vi "Handle setConfiguration.vi"(8 "error in (no error)":errorcluster, 10 "setConfiguration":variant, 11 "Inst.RP100 in":refnum<class "Inst.RP100.lvclass">) -> (0 "error out":errorcluster, 3 "Inst.RP100 out":refnum<class "Inst.RP100.lvclass">)   [LabVIEW 2019, in "Inst.RP100.lvclass"]
uses:
  Inst.RP100.lvclass
  45e4b271-6884-462c-ad3a-d505ab08eb62.vi
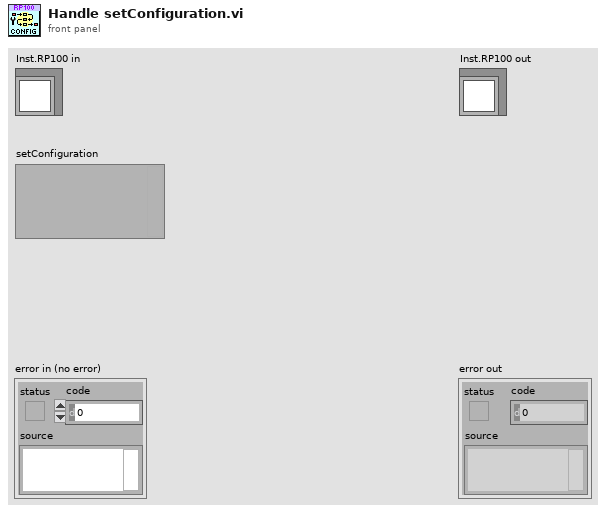
[diagram p1: front panel]
types:
  T1 = typedef "Inst.RP100.lvclass/Inst.RP100.Configuration--Cluster.ctl" = cluster{"Example Setting 1":dbl, "Example Setting 2":dbl, "Example Setting 3":string}
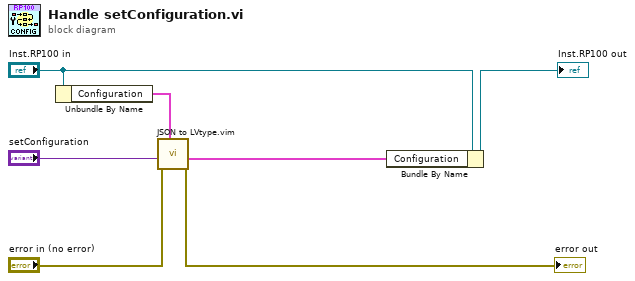
[diagram p0: block diagram]
diagram:
  n1 = Unbundle By Name("Inst.RP100 in") -> ("Configuration"=w6:T1)
  n2 = call "JSON to LVtype.vim"("type"=w6, "error in (no error)"="error in (no error)", "JSON Data in"="setConfiguration") -> ("error out"=→"error out":errorcluster, "Data out"=w1:T1)  [unwired: 7 in]
  n3 = Bundle By Name(cluster="Inst.RP100 in", "Configuration"=w1) -> (→"Inst.RP100 out":refnum<class "Inst.RP100.lvclass">)
